vi "Generate Address API.vi"(8 "error in (no error)":errorcluster, 11 "DVR IN":refnum<data-value>) -> (0 "error out":errorcluster, 3 "DVR OUT":refnum<data-value>)   [LabVIEW 2020, in "Addressing Mode.lvclass"]
uses:
  Addressing Mode.lvclass
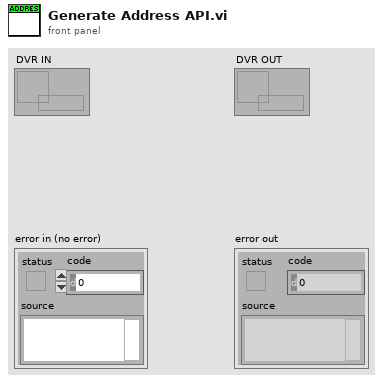
[diagram p1: front panel]
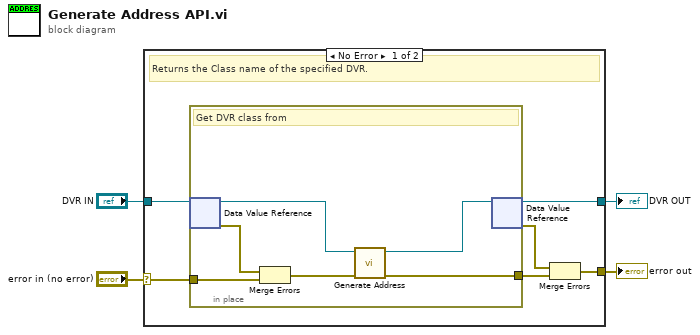
[diagram p0: block diagram]
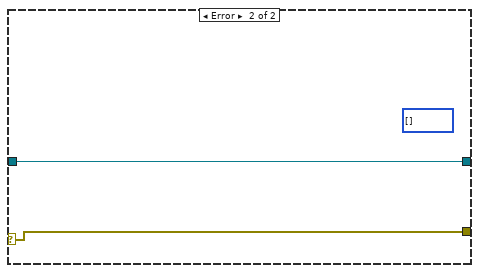
[diagram p2: hidden frame]
diagram:
  n1 = case shown="No Error" "error in (no error)" {
    selector: "error in (no error)" -> [w10 w18]
    tunnel: [w8 w18] -> w3
    tunnel: "DVR IN" -> [w6 w17]
    tunnel: [w5 w17] -> w1
    frame No Error {
      # "Returns the Class name of the specified DVR."
      n2 = in-place {
        in-place-border: w10 -> [w16]
        in-place-border: [w13] -> w7
        # "Get DVR class from"
        n3 = in-place-dvr #1(w6) -> (w12:refnum<class "Addressing Mode.lvclass">, w15:errorcluster)
        n4 = Merge Errors(w15, w16) -> (w14:errorcluster)
        n5 = call-dynamic "Generate Address.vi"("error in (no error)"=w14, "Addressing Mode in"=w12) -> ("error out"=w13:errorcluster, "Addressing Mode out"=w11:refnum<class "Addressing Mode.lvclass">)  [unwired: 8 in]
        n6 = in-place-dvr #1(w11) -> (w5:refnum<data-value>, w9:errorcluster)
      }
      n7 = Merge Errors(w9, w7) -> (w8:errorcluster)
    }
    frame Error {
      (unwired) i16[] [] ("Address")
    }
  }
  "error out" <- w3
  "DVR OUT" <- w1
